vi "Teleop.vi"(10 "Match Info":T2={"Autonomous Elapsed Seconds"=0.0, "TeleOp Elapsed Seconds"=59.421, "Disabled Elapsed Seconds"=50.178, "Visited Autonomous"=FALSE, "Visited TeleOp"=TRUE, "Visited Disabled"=TRUE, "Autonomous Settings"={"Autonomous Style"=enum."Independent", "VI Refnum"=refnum}}, 11 "Call Context":T3=enum."Stop") -> ()   [LabVIEW 2014]
doc: "This VI is called for each TeleOp packet received from the DS where the robot is not disabled. It is often used to read from the joysticks and update I/O or to update setpoints for timed control loops. It should complete and return within 20 milliseconds or it may miss DS packets."
uses:
  <vilib>/Rock Robotics/WPI/DriverStation/WPI_DriverStationDerivedRobotMode.ctl
  <vilib>/Rock Robotics/WPI/DriverStation/WPI_DriverStationMatch Info.ctl
  <vilib>/Rock Robotics/WPI/RobotDrive/WPI_RobotDriveGetSetRefNum.vi
  <vilib>/Rock Robotics/WPI/Joystick/WPI_JoystickGetSetRefNum.vi
  <vilib>/Rock Robotics/Network Tables/SD Write Numeric Array.vi
  <vilib>/Rock Robotics/Network Tables/SD Write Boolean Array.vi
  Robot Global Data.vi
  <vilib>/Rock Robotics/WPI/RobotDrive/WPI_RobotDriveMecanumDrive_Cartesian.vi
panel:
  out "current (A)":dbl(graph)
  in  "Clear Sticky Faults":bool
  in  "PID gains":T1={"proportional gain (Kc)"=0.021, "integral time (Ti, min)"=0.0, "derivative time (Td, min)"=0.0} {"derivative time (Td, min)" format="%.3f"; "integral time (Ti, min)" format="%.3f"; "proportional gain (Kc)" format="%.3f"}
  # "EDITED: 3/8/15"
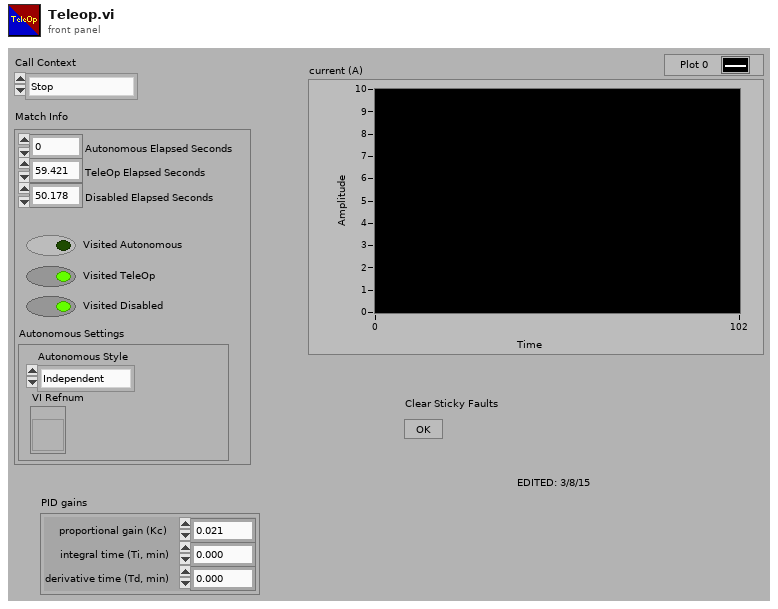
[diagram p1: front panel]
types:
  T1 = cluster{"proportional gain (Kc)":dbl, "integral time (Ti, min)":dbl, "derivative time (Td, min)":dbl}
  T2 = typedef "WPI_DriverStationMatch Info.ctl" = cluster{"Autonomous Elapsed Seconds":dbl, "TeleOp Elapsed Seconds":dbl, "Disabled Elapsed Seconds":dbl, "Visited Autonomous":bool, "Visited TeleOp":bool, "Visited Disabled":bool, "Autonomous Settings":cluster{"Autonomous Style":enum16{"Iterative", "Independent"}, "VI Refnum":refnum<vi>}}
  T3 = typedef "WPI_DriverStationDerivedRobotMode.ctl" = enum16{"Init", "Execute", "Stop"}
  T4 = typedef "WPI_JoystickDevRef.ctl" = cluster{"Device":T5}
  T5 = typedef "WPI_JoystickDeviceEnum.ctl" = enum16{"USB 0", "USB 1", "USB 2", "USB 3", "USB 4", "USB 5"}
  T6 = typedef "WPI_RobotDriveDevRef.ctl" = cluster{"DevStatus":errorcluster, "Motors[]":T7[], "Square Inputs":bool, "Max Output":dbl}
  T7 = typedef "WPI_MotorControlDeviceRef.ctl" = cluster{"DeviceStatus":errorcluster, "Type":T8, "PWM":cluster{"Controller":T9, "PWM Channel":T10, "DeadBand":T11}, "CAN":cluster{"Device Number":u8, "Control Mode":T12, "Semaphore":T13, "Max Vout":dbl, "TalonSRX Control Mode":T14}, "Invert":bool, "TransformRef":T15, "InvTransformRef":T15}
  T8 = typedef "WPI_MotorControlType.ctl" = enum16{"PWM", "CAN", "CANTalonSRX"}
  T9 = typedef "FPGA_TypedefDigitalModule.ctl" = enum16{"Controller 1"}
  T10 = typedef "FPGA_DIOPWMChannel.ctl" = enum8{"PWM 0", "PWM 1", "PWM 2", "PWM 3", "PWM 4", "PWM 5", "PWM 6", "PWM 7", "PWM 8", "PWM 9", "PWM MXP 0", "PWM MXP 1", "PWM MXP 2", "PWM MXP 3", "PWM MXP 4", "PWM MXP 5", "PWM MXP 6", "PWM MXP 7", "PWM MXP 8", "PWM MXP 9", "Invalid"}
  T11 = typedef "WPI_PWMDeadband.ctl" = cluster{"Name":string, "maxPositivePwm":i32, "minPositivePwm":i32, "centerPwm":i32, "maxNegativePwm":i32, "minNegativePwm":i32, "angularRange":u16}
  T12 = typedef "WPI_CANJaguar_ControlMode.ctl" = enum8{"Percent VBus", "Current", "Speed", "Position", "Voltage"}
  T13 = typedef "Semaphore RefNum" = refnum<k1>
  T14 = typedef "WPI_CANTalonSRX_APIControlMode.ctl" = enum8{"Percent VBus", "Speed", "Position", "Slave", "Unchanged / Invalid"}
  T15 = typedef "WPI_PWMTransform_ConPane.ctl" = refnum<vi>
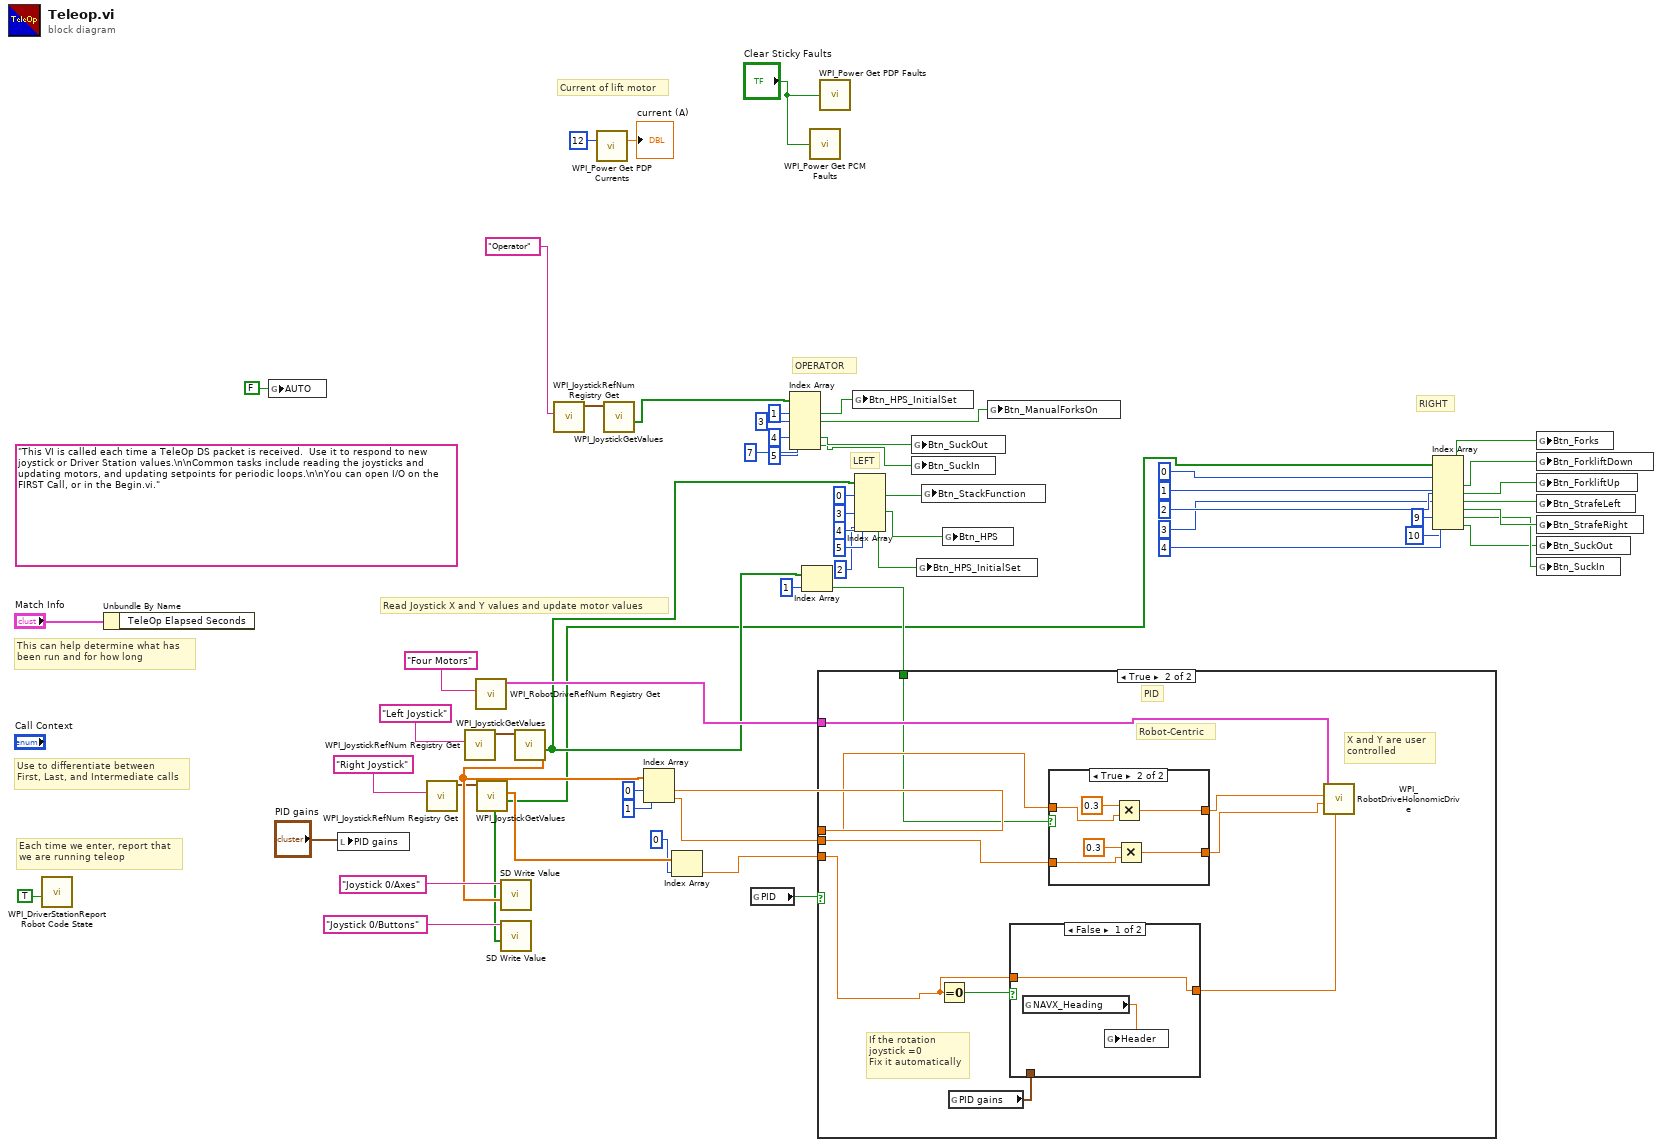
[diagram p0: block diagram]
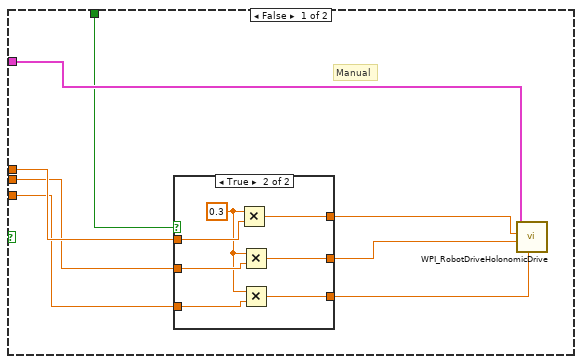
[diagram p2: hidden frame]
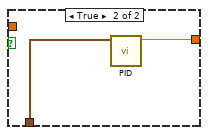
[diagram p4: hidden frame]
diagram:
  (unwired) "This VI is called each time a TeleOp DS packet is received.  Use it to respond to new joystick or Driver Station values.\n\nCommon tasks include reading the joysticks and updating motors, and updating setpoints for periodic loops.\n\nYou can open I/O on the FIRST Call, or in the Begin.vi."
  # "LEFT"
  # "OPERATOR"
  # "RIGHT"
  # "Current of lift motor"
  # "Each time we enter, report that\nwe are running teleop"
  # "Use to differentiate between\nFirst, Last, and Intermediate calls"
  # "This can help determine what has\nbeen run and for how long"
  # "Read Joystick X and Y values and update motor values"
  n1 = call <vilib>:"WPI_DriverStationReport Robot Code State.vi"("TeleOp"=TRUE ("Autonomous")) -> ()  [unwired: 10 in, 1 out]
  n2 = Unbundle By Name("Match Info") -> ()  [unwired: 1 out]
  n3 = global write "Robot Global Data.vi" "AUTO"(FALSE ("AUTO")) -> ()
  n4 = local write "PID gains"("PID gains") -> ()
  n5 = call <vilib>:"WPI_JoystickRefNum Registry Get.vi"("refnum name"="Right Joystick") -> ("JoystickDevRef"=w47:T4)  [unwired: 1 in, 9 out]
  n6 = call <vilib>:"WPI_JoystickRefNum Registry Get.vi"("refnum name"="Left Joystick") -> ("JoystickDevRef"=w59:T4)  [unwired: 1 in, 9 out]
  n7 = call <vilib>:"WPI_RobotDriveRefNum Registry Get.vi"("refnum name"="Four Motors") -> ("RobotDriveDevRef"=w48:T6)  [unwired: 1 in, 9 out]
  n8 = call <vilib>:"WPI_JoystickGetValues.vi"("JoystickDevRef"=w47) -> ("Buttons"=w19:bool[], "Axes"=w45:dbl[])  [unwired: 6 in, 3 out]
  n9 = call-poly <vilib>:"SD Write Value.vi"("Boolean Array"=w19, "Name"="Joystick 0/Buttons") -> ()  [unwired: 8 in, 2 out]
  n10 = call <vilib>:"WPI_JoystickGetValues.vi"("JoystickDevRef"=w59) -> ("Buttons"=w40:bool[], "Axes"=w53:dbl[])  [unwired: 6 in, 3 out]
  n11 = call-poly <vilib>:"SD Write Value.vi"("Numeric Array"=w53, "Name"="Joystick 0/Axes") -> ()  [unwired: 8 in, 2 out]
  n12 = call <vilib>:"WPI_JoystickRefNum Registry Get.vi"("refnum name"="Operator") -> ("JoystickDevRef"=w22:T4)  [unwired: 1 in, 9 out]
  n13 = call <vilib>:"WPI_Power Get PDP Currents.vi"("PDP Channel"=12) -> ("current (A)"=→"current (A)":dbl)  [unwired: 12 in, 2 out]
  n14 = call <vilib>:"WPI_JoystickGetValues.vi"("JoystickDevRef"=w22) -> ("Buttons"=w20:bool[])  [unwired: 6 in, 4 out]
  n15 = Index Array(array=w53, index #1=0 ("index"), index #2=1 ("index")) -> (element #1=w50:dbl, element #2=w49:dbl)
  n16 = Index Array(array=w45, index=0) -> (element=w43:dbl)
  n17 = global read "Robot Global Data.vi" "PID"() -> (w1:bool)
  n18 = Index Array(array=w20, index #1=1 ("index"), index #2=3 ("index"), index #3=7 ("index"), index #4=4 ("index"), index #5=5 ("index")) -> (element #1=w16:bool, element #2=w15:bool, element #4=w5:bool, element #5=w4:bool)  [unwired: 1 out]
  n19 = Index Array(array=w40, index=1) -> (element=w41:bool)
  n20 = call <vilib>:"WPI_Power Get PCM Faults.vi"("Clear Sticky Faults"="Clear Sticky Faults") -> ()  [unwired: 11 in, 4 out]
  n21 = case shown="True" w1 {
    tunnel: w50 -> [w70 w90]
    tunnel: w49 -> [w69 w89]
    tunnel: w43 -> [w65 w82]
    tunnel: w48 -> [w68 w88]
    tunnel: w41 -> [w63 w87]
    frame False {
      # "Manual"
      n22 = case shown="True" w63 {
        tunnel: [w73 w80] -> w67
        tunnel: [w72 w79] -> w66
        tunnel: w70 -> [w73 w78]
        tunnel: w69 -> [w72 w77]
        tunnel: w65 -> [w71 w76]
        tunnel: [w71 w75] -> w64
        frame False {
        }
        frame True {
          w74 = 0.3 ("x")
          n23 = Multiply(x=w74, y=w78) -> (x*y=w80:dbl)
          n24 = Multiply(x=w74, y=w77) -> (x*y=w79:dbl)
          n25 = Multiply(x=w74, y=w76) -> (x*y=w75:dbl)
        }
      }
      n26 = call-poly <vilib>:"WPI_RobotDriveHolonomicDrive.vi"("Rotation"=w64, "Y"=w66, "X"=w67, "RobotDriveDevRef"=w68) -> ()  [unwired: 5 in, 3 out]
    }
    frame True {
      # "If the rotation\njoystick =0\nFix it automatically"
      # "X and Y are user \ncontrolled"
      # "Robot-Centric"
      # "PID"
      n27 = Equal To 0?(x=w82) -> (x = 0?=w83:bool)
      n28 = global read "Robot Global Data.vi" "PID gains"() -> (w81:T1)
      n29 = case shown="False" w83 {
        tunnel: [w92 w94] -> w86
        tunnel: w82 -> [w92 _]
        tunnel: w81 -> [_ w93]
        frame False {
          n30 = global read "Robot Global Data.vi" "NAVX_Heading"() -> (w91:dbl)
          n31 = global write "Robot Global Data.vi" "Header"(w91) -> ()
        }
        frame True {
          n32 = call "PID.vi"("PID gains"=w93) -> ("output"=w94:dbl)  [unwired: 10 in]
        }
      }
      n33 = case shown="True" w87 {
        tunnel: [w96 w100] -> w85
        tunnel: [w95 w99] -> w84
        tunnel: w90 -> [w96 w98]
        tunnel: w89 -> [w95 w97]
        frame False {
        }
        frame True {
          n34 = Multiply(x=0.3, y=w98) -> (x*y=w100:dbl)
          n35 = Multiply(x=0.3, y=w97) -> (x*y=w99:dbl)
        }
      }
      n36 = call-poly <vilib>:"WPI_RobotDriveHolonomicDrive.vi"("Rotation"=w86, "Y"=w84, "X"=w85, "RobotDriveDevRef"=w88) -> ()  [unwired: 5 in, 3 out]
    }
  }
  n37 = call <vilib>:"WPI_Power Get PDP Faults.vi"("Clear Sticky Faults"="Clear Sticky Faults") -> ()  [unwired: 10 in, 5 out]
  n38 = global write "Robot Global Data.vi" "Btn_HPS_InitialSet"(w16) -> ()
  n39 = Index Array(array=w40, index #1=0 ("index"), index #2=3 ("index"), index #3=4 ("index"), index #4=5 ("index"), index #5=2 ("index")) -> (element #1=w38:bool, element #3=w24:bool, element #5=w8:bool)  [unwired: 2 out]
  n40 = global write "Robot Global Data.vi" "Btn_SuckOut"(w5) -> ()
  n41 = global write "Robot Global Data.vi" "Btn_SuckIn"(w4) -> ()
  n42 = global write "Robot Global Data.vi" "Btn_HPS_InitialSet"(w8) -> ()
  n43 = global write "Robot Global Data.vi" "Btn_StackFunction"(w38) -> ()
  n44 = global write "Robot Global Data.vi" "Btn_HPS"(w24) -> ()
  n45 = global write "Robot Global Data.vi" "Btn_ManualForksOn"(w15) -> ()
  n46 = Index Array(array=w19, index #1=0 ("index"), index #2=1 ("index"), index #3=2 ("index"), index #4=3 ("index"), index #5=4 ("index"), index #6=9 ("index"), index #7=10 ("index")) -> (element #1=w37:bool, element #2=w33:bool, element #3=w32:bool, element #4=w30:bool, element #5=w29:bool, element #6=w12:bool, element #7=w11:bool)
  n47 = global write "Robot Global Data.vi" "Btn_Forks"(w37) -> ()
  n48 = global write "Robot Global Data.vi" "Btn_ForkliftDown"(w33) -> ()
  n49 = global write "Robot Global Data.vi" "Btn_ForkliftUp"(w32) -> ()
  n50 = global write "Robot Global Data.vi" "Btn_StrafeLeft"(w30) -> ()
  n51 = global write "Robot Global Data.vi" "Btn_StrafeRight"(w29) -> ()
  n52 = global write "Robot Global Data.vi" "Btn_SuckOut"(w11) -> ()
  n53 = global write "Robot Global Data.vi" "Btn_SuckIn"(w12) -> ()
